vi "Analyze Blobs.vi"(0 "Image In":T2, 1 "Blob Data":T3) -> (7 "Image Out":T2, 8 "Target Data":T1)   [LabVIEW 2015]
uses:
  <vilib>/vision/Image Controls.llb/IMAQ Image.ctl
  <vilib>/Analysis/Matrix/Datatypes/RealMatrix.ctl
  <vilib>/Analysis/coordinate.llb/Euler Rotation Order.ctl
  <vilib>/Analysis/baseanly.llb/A x Vector.vi
  <vilib>/Analysis/coordinate.llb/3D Cartesian Coordinate Rotation (Euler) (Scalar).vi
  <vilib>/Analysis/baseanly.llb/Real Inverse Matrix.vi
  <vilib>/Rock Robotics/Network Tables/NT Write Number.vi
  <vilib>/Analysis/NI_AALBase.lvlib
  <vilib>/Analysis/Matrix/NI_Matrix.lvlib
  <vilib>/Analysis/NI_AALPro.lvlib
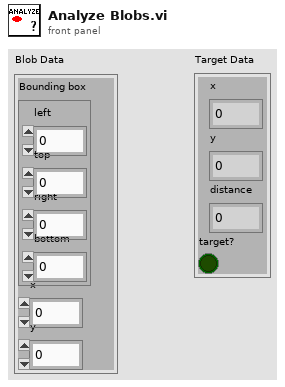
[diagram p1: front panel]
types:
  T1 = cluster{"x":dbl, "y":dbl, "distance":dbl, "target?":bool}
  T2 = typedef "IMAQ Image.ctl" = refnum<image>
  T3 = cluster{"Bounding box":cluster{"left":dbl, "top":dbl, "right":dbl, "bottom":dbl}, "x":dbl, "y":dbl}
  T4 = typedef "ROI Descriptor" = cluster{"Global Rectangle":i32[], "Contours":cluster{"ID":enum32{"External", "Internal"}, "Type":u32, "Coordinates":i32[]}[]}
  T5 = typedef "Edge New.ctl" = cluster{"Location (Pixel)":cluster{"X":sgl, "Y":sgl}, "Location (Real-World)":cluster{"X":sgl, "Y":sgl}, "Distance (Pixel)":dbl, "Distance (Real-World)":dbl, "Strength":dbl, "Noise":dbl, "Rising?":bool}
  T6 = typedef "NI_Matrix.lvlib/RealMatrix.ctl" = dbl[][]
  T7 = typedef "NI_AALPro.lvlib/Euler Rotation Order.ctl" = u16
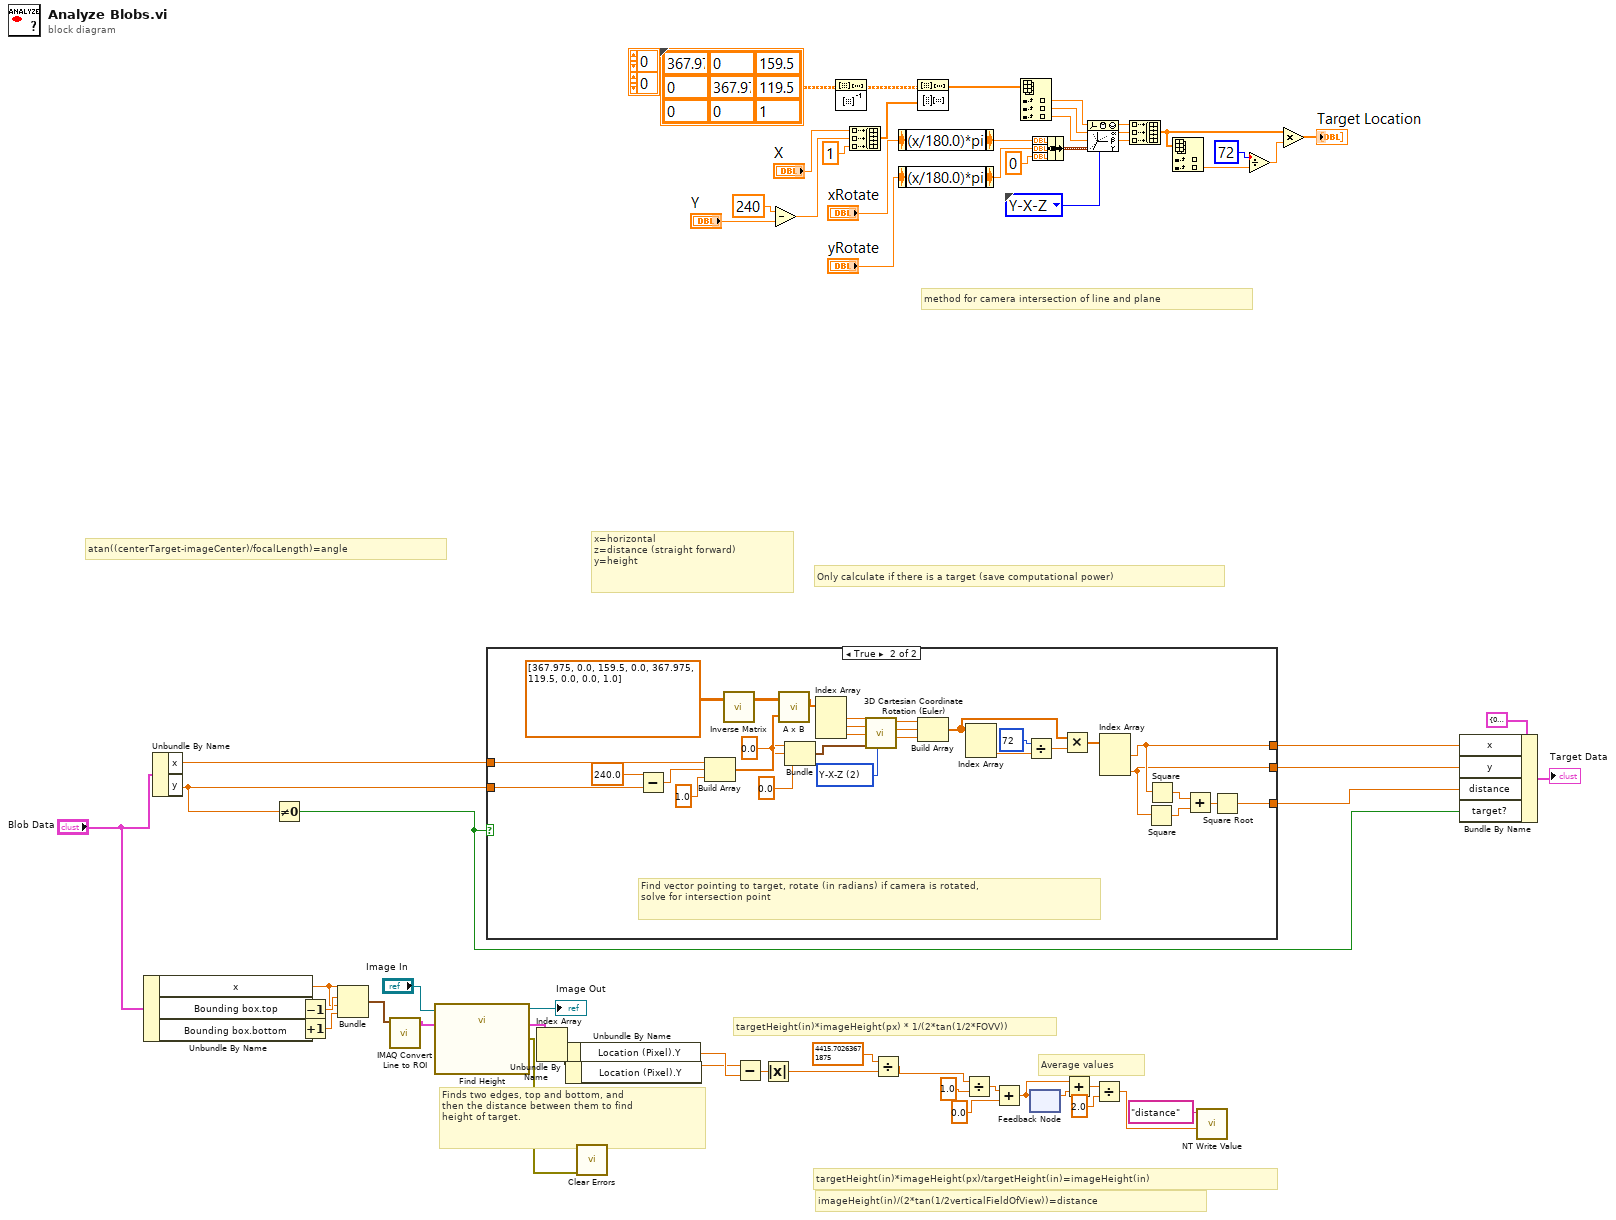
[diagram p0: block diagram]
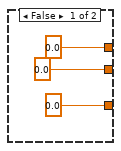
[diagram p2: hidden frame]
diagram:
  # "Only calculate if there is a target (save computational power)"
  # "method for camera intersection of line and plane"
  # "targetHeight(in)*imageHeight(px) * 1/(2*tan(1/2*FOVV))"
  # "x=horizontal\nz=distance (straight forward) \ny=height"
  # "atan((centerTarget-imageCenter)/focalLength)=angle"
  # "Finds two edges, top and bottom, and\nthen the distance between them to find\nheight of target."
  # "imageHeight(in)/(2*tan(1/2verticalFieldOfView))=distance"
  # "targetHeight(in)*imageHeight(px)/targetHeight(in)=imageHeight(in)"
  # "Average values"
  n1 = Unbundle By Name("Blob Data") -> ("x"=w24:dbl, "Bounding box.top"=w26:dbl, "Bounding box.bottom"=w23:dbl)
  n2 = Unbundle By Name("Blob Data") -> ("x"=w7:dbl, "y"=w6:dbl)
  n3 = Not Equal To 0?(x=w6) -> (x != 0?=w2:bool)
  n4 = Decrement(x=w26) -> (x-1=w25:dbl)
  n5 = Increment(x=w23) -> (x+1=w22:dbl)
  n6 = Bundle("x"=w24, w25, "x"=w24, w22) -> (w21:cluster{"x":dbl, dbl, "x":dbl, dbl})  [unwired: 1 in]
  n7 = call "IMAQ Convert Line to ROI"("Line"=w21) -> ("ROI Descriptor"=w30:T4)  [unwired: 8 in, 1 out]
  n8 = call "Find Height"("Image In"="Image In", "ROI Descriptor (Edge Detector 1)"=w30) -> ("Image Out"=→"Image Out":T2, "Edge Information (Edge Detector 1)"=w29:T5[], "error out"=w11:errorcluster)  [unwired: 23 in]
  n9 = case shown="True" w2 {
    tunnel: w7 -> [_ w69]
    tunnel: w6 -> [_ w50]
    tunnel: [0.0 w44] -> w5
    tunnel: [0.0 w43] -> w4
    tunnel: [0.0 w42] -> w3
    frame False {
    }
    frame True {
      w41 = 0.0 ("x-y")
      w58 = T7 2 items=["X-Y-Z", "X-Z-Y", "Y-X-Z", "Y-Z-X", "Z-X-Y", "Z-Y-X", "X-Y-X", "X-Z-X", "Y-X-Y", "Y-Z-Y", "Z-X-Z", "Z-Y-Z"] ("rotation order")
      # "Find vector pointing to target, rotate (in radians) if camera is rotated,\nsolve for intersection point"
      n10 = Subtract(x=240.0 ("element"), y=w50) -> (x-y=w51:dbl)
      n11 = Build Array(w69, w51, 1.0 ("element")) -> (w66:dbl[])
      n12 = call-poly <vilib>:"Inverse Matrix.vi"("Input Matrix"=T6 [[367.975, 0.0, 159.5], [0.0, 367.975, 119.5], [0.0, 0.0, 1.0]]) -> ("Inverse Matrix"=w67:T6)  [unwired: 1 in, 1 out]
      n13 = call-poly <vilib>:"A x B.vi"("Vector"=w66, "A"=w67) -> ("A x Vector"=w65:dbl[])  [unwired: 1 out]
      n14 = Bundle("x-y"=w41, "x-y"=w41, "x-y"=0.0) -> (w52:cluster{"x-y":dbl, "x-y":dbl, "x-y":dbl})  [unwired: 1 in]
      n15 = Index Array(array=w65) -> (element #1=w59:dbl, element #2=w60:dbl, element #3=w61:dbl)  [unwired: 3 in]
      n16 = call-poly <vilib>:"3D Cartesian Coordinate Rotation (Euler).vi"("rotation order"=w58, "Euler Angles"=w52, "z"=w61, "y"=w60, "x"=w59) -> ("z out"=w64:dbl, "y out"=w63:dbl, "x out"=w62:dbl)  [unwired: 3 in, 1 out]
      n17 = Build Array(w62, w63, w64) -> (w54:dbl[])
      n18 = Index Array(array=w54) -> (element #2=w56:dbl)  [unwired: 2 in, 1 out]
      n19 = Divide(x=72 ("y"), y=w56) -> (x/y=w55:dbl)
      n20 = Multiply ("Multiply.vi")(x=w54, y=w55) -> (x*y=w48:dbl[])
      n21 = Index Array(array=w48) -> (element #1=w44:dbl, element #3=w43:dbl)  [unwired: 3 in, 1 out]
      n22 = Square(x=w43) -> (x^2=w46:dbl)
      n23 = Square(x=w44) -> (x^2=w45:dbl)
      n24 = Add(x=w45, y=w46) -> (x+y=w47:dbl)
      n25 = Square Root(x=w47) -> (sqrt(x)=w42:dbl)
    }
  }
  n26 = Index Array(array=w29) -> (element #1=w19:T5, element #2=w18:T5)  [unwired: 2 in]
  n27 = Unbundle By Name(w19) -> ("Location (Pixel).Y"=w17:sgl)
  n28 = Unbundle By Name(w18) -> ("Location (Pixel).Y"=w16:sgl)
  n29 = call <vilib>:"Clear Errors.vi"("error in (no error)"=w11) -> ()  [unwired: 5 in, 2 out]
  n30 = Subtract(x=w16, y=w17) -> (x-y=w15:sgl)
  n31 = Absolute Value(x=w15) -> (abs(x)=w9:sgl)
  n32 = Divide ("FOV inches")(x=sgl 4415.7026, y=w9) -> (x/y=w10:sgl)
  n33 = Divide ("FOV inches")(x=w10, y=1.0) -> (x/y=w36:dbl)
  n34 = Add(x=w36, y=0.0) -> (x+y=w33:dbl)
  n35 = feedback #1() -> (w34:dbl)  [unwired: 1 in]
  n36 = feedback-in #1(w33) -> ()
  n37 = Add(x=w33, y=w34) -> (x+y=w32:dbl)
  n38 = Divide ("FOV inches")(x=w32, y=2.0) -> (x/y=w28:dbl)
  n39 = call-poly <vilib>:"NT Write Value.vi"("Numeric"=w28, "Name"="distance") -> ()  [unwired: 9 in, 1 out]
  n40 = Bundle By Name(cluster=T1 {"x"=0.0, "y"=0.0, "distance"=0.0, "target?"=FALSE} ("input cluster"), "x"=w5, "y"=w4, "distance"=w3, "target?"=w2) -> (→"Target Data":T1)
